vi "MotionDoneAll.vi"(8 "StepError":errorcluster caption="StepError）", 9 "PicError":errorcluster, 10 "com in":refnum<visa-resource-name>, 11 "CmdLib In":refnum<k24>) -> (0 "StepErrorOut":errorcluster, 1 "PicErrorOut":errorcluster, 2 "com out":refnum<visa-resource-name>, 3 "CmdLib Out":refnum<k24>, 4 "执行":bool)   [LabVIEW 2018]
uses:
  Device VIs/CmdLib.dll
  Device VIs/Verbal.vi
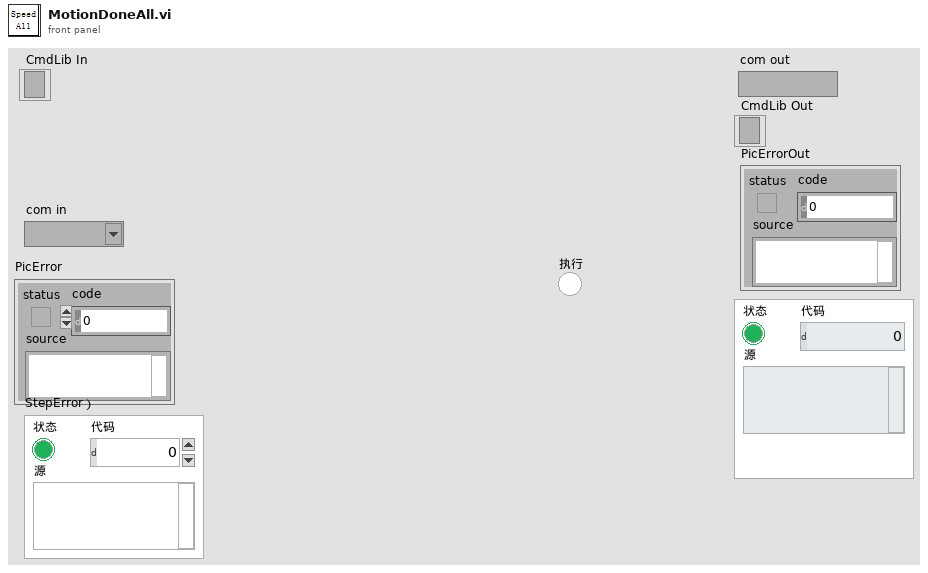
[diagram p1: front panel]
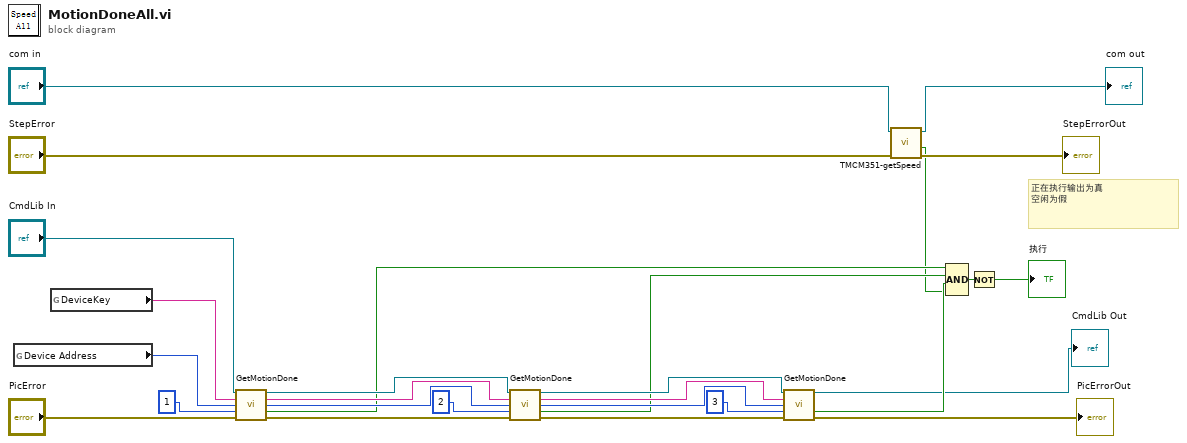
[diagram p0: block diagram]
diagram:
  # "正在执行输出为真\n空闲为假"
  n1 = global read "Verbal.vi" "Device Address"() -> (w16:i32)
  n2 = global read "Verbal.vi" "DeviceKey"() -> (w17:string)
  n3 = call "GetMotionDone.vi"("CmdLib In"="CmdLib In", "DeviceKey In"=w17, "Device Address In"=w16, "Motor"=1, "error in (no error)"="PicError") -> ("CmdLib Out"=w27:refnum<k24>, "DeviceKey Out"=w23:string, "Device Address Out"=w22:i32, "Is Motion Done"=w8:bool, "error out"=w26:errorcluster)  [unwired: 6 in]
  n4 = call "GetMotionDone.vi"("CmdLib In"=w27, "DeviceKey In"=w23, "Device Address In"=w22, "Motor"=2, "error in (no error)"=w26) -> ("CmdLib Out"=w25:refnum<k24>, "DeviceKey Out"=w21:string, "Device Address Out"=w20:i32, "Is Motion Done"=w7:bool, "error out"=w24:errorcluster)  [unwired: 6 in]
  n5 = call "GetMotionDone.vi"("CmdLib In"=w25, "DeviceKey In"=w21, "Device Address In"=w20, "Motor"=3, "error in (no error)"=w24) -> ("CmdLib Out"=→"CmdLib Out":refnum<k24>, "Is Motion Done"=w6:bool, "error out"=→"PicErrorOut":errorcluster)  [unwired: 6 in, 2 out]
  n6 = call "TMCM351-getSpeed.vi"("错误输入"="StepError", "com in"="com in") -> ("错误输出"=→"StepErrorOut":errorcluster, "Motion Done"=w5:bool, "com out"=→"com out":refnum<visa-resource-name>)  [unwired: 2 in, 1 out]
  n7 = Compound Arithmetic op=AND ("复合运算")(w8, w7, w6, w5) -> (w4:bool)
  n8 = Not(x=w4) -> (.not. x?=→"执行":bool)
